vi "IntakeTeleopCommand.vi"(11 "Buttons":bool[](array[boolean])) -> ()   [LabVIEW 2017]
uses:
  IntakeCommand.ctl
  RunMode.ctl
  Robot Global Data.vi
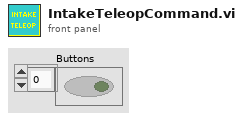
[diagram p1: front panel]
types:
  T1 = typedef "RunMode.ctl" = enum16{"Auto", "Teleop", "Disabled"}
  T2 = typedef "IntakeCommand.ctl" = cluster{"Collect":bool, "Deposit":bool, "Mode":T1}
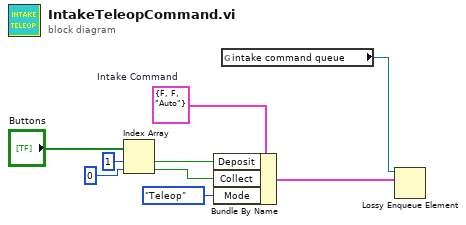
[diagram p0: block diagram]
diagram:
  w2 = T2 {"Collect"=FALSE, "Deposit"=FALSE, "Mode"=enum."Auto"}  # Intake Command
  n1 = Index Array(array="Buttons", index #1=1 ("index"), index #2=0 ("index")) -> (element #1=w6:bool, element #2=w7:bool)
  n2 = Bundle By Name(cluster=w2, "Deposit"=w6, "Collect"=w7, "Mode"=RunMode."Teleop") -> (w4:T2)
  n3 = global read "Robot Global Data.vi" "intake command queue"() -> (w1:refnum<queue>)
  n4 = Lossy Enqueue Element(queue=w1, element=w4) -> ()  [unwired: 1 in, 4 out]
